vi "CrossHair Calc.vi"   [LabVIEW 2012]
types:
  T1 = typedef "WPI_ServoDeviceRef.ctl" = cluster{"DeviceStatus":errorcluster, "Digital Module":T2, "PWM Channel":T3, "DeadBand":T4}
  T2 = typedef "FPGA_TypedefDigitalModule.ctl" = enum16{"Digital Module 1", "Digital Module 2"}
  T3 = typedef "FPGA_DIOPWMChannel.ctl" = enum8{"PWM 1", "PWM 2", "PWM 3", "PWM 4", "PWM 5", "PWM 6", "PWM 7", "PWM 8", "PWM 9", "PWM 10", "Invalid"}
  T4 = typedef "WPI_PWMDeadband.ctl" = cluster{"Name":string, "maxPositivePwm":i32, "minPositivePwm":i32, "centerPwm":i32, "maxNegativePwm":i32, "minNegativePwm":i32, "angularRange":u16}
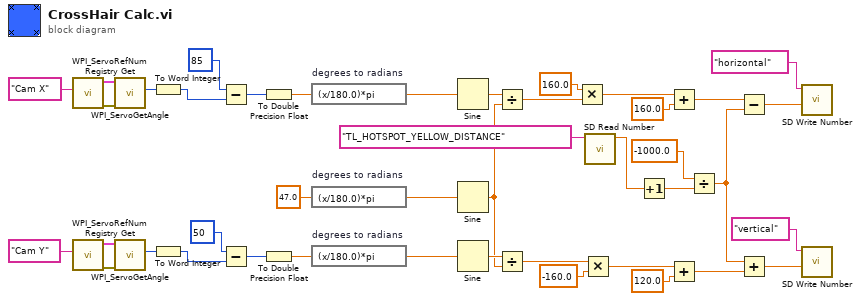
[diagram p0: block diagram]
diagram:
  n1 = call <vilib>:"WPI_ServoRefNum Registry Get.vi"("refnum name"="Cam X") -> ("error out"=w41:errorcluster, "ServoDeviceRef"=w42:T1)  [unwired: 9 in]
  n2 = call <vilib>:"WPI_ServoRefNum Registry Get.vi"("refnum name"="Cam Y") -> ("error out"=w38:errorcluster, "ServoDeviceRef"=w39:T1)  [unwired: 9 in]
  n3 = call <vilib>:"WPI_ServoGetAngle.vi"("ServoDeviceRef"=w42, "error in (no error)"=w41) -> ("Angle"=w35:u16)  [unwired: 6 in, 2 out]
  n4 = call <vilib>:"WPI_ServoGetAngle.vi"("ServoDeviceRef"=w39, "error in (no error)"=w38) -> ("Angle"=w36:u16)  [unwired: 6 in, 2 out]
  n5 = To Word Integer(number=w35) -> (16bit integer=w1:i16)
  n6 = To Word Integer(number=w36) -> (16bit integer=w3:i16)
  n7 = Subtract(x=i16 85 ("y"), y=w1) -> (x-y=w11:i16)
  n8 = Subtract(x=i16 50 ("y"), y=w3) -> (x-y=w13:i16)
  n9 = To Double Precision Float(number=w11) -> (double precision float=w10:dbl)
  n10 = To Double Precision Float(number=w13) -> (double precision float=w12:dbl)
  n11 = expression code="(x/180.0)*pi" "degrees to radians"(w10) -> (w26:dbl)
  n12 = expression code="(x/180.0)*pi" "degrees to radians"(47.0) -> (w29:dbl)
  n13 = expression code="(x/180.0)*pi" "degrees to radians"(w12) -> (w30:dbl)
  n14 = Sine(x=w26) -> (sin(x)=w25:dbl)
  n15 = Sine(x=w29) -> (sin(x)=w24:dbl)
  n16 = Sine(x=w30) -> (sin(x)=w27:dbl)
  n17 = Divide(x=w25, y=w24) -> (x/y=w22:dbl)
  n18 = Divide(x=w27, y=w24) -> (x/y=w23:dbl)
  n19 = Multiply(x=160.0, y=w22) -> (x*y=w19:dbl)
  n20 = Multiply(x=w23, y=-160.0) -> (x*y=w17:dbl)
  n21 = call <vilib>:"SD Read Number.vi"("Name"="TL_HOTSPOT_YELLOW_DISTANCE") -> ("Numeric"=w31:dbl)  [unwired: 8 in, 2 out]
  n22 = Increment(x=w31) -> (x+1=w32:dbl)
  n23 = Add(x=w19, y=160.0) -> (x+y=w6:dbl)
  n24 = Add(x=w17, y=120.0) -> (x+y=w9:dbl)
  n25 = Divide(x=-1000.0 ("y"), y=w32) -> (x/y=w7:dbl)
  n26 = Subtract(x=w6, y=w7) -> (x-y=w5:dbl)
  n27 = Add(x=w7, y=w9) -> (x+y=w8:dbl)
  n28 = call <vilib>:"SD Write Number.vi"("Numeric"=w5, "Name"="horizontal") -> ()  [unwired: 8 in, 2 out]
  n29 = call <vilib>:"SD Write Number.vi"("Numeric"=w8, "Name"="vertical") -> ()  [unwired: 8 in, 2 out]
